vi "NumIntegrate_Rk4_K_Dbl.vi"(11 "input matrix":T1) -> (3 "output matrix":T1)   [LabVIEW 2019]
doc: "NOT DONE"
uses:
  <vilib>/Analysis/Matrix/Datatypes/RealMatrix.ctl
  <vilib>/Analysis/Matrix/NI_Matrix.lvlib
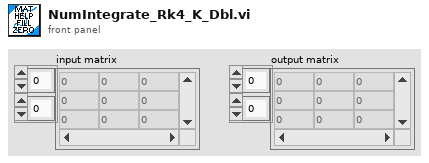
[diagram p1: front panel]
types:
  T1 = typedef "NI_Matrix.lvlib/RealMatrix.ctl" = dbl[][]
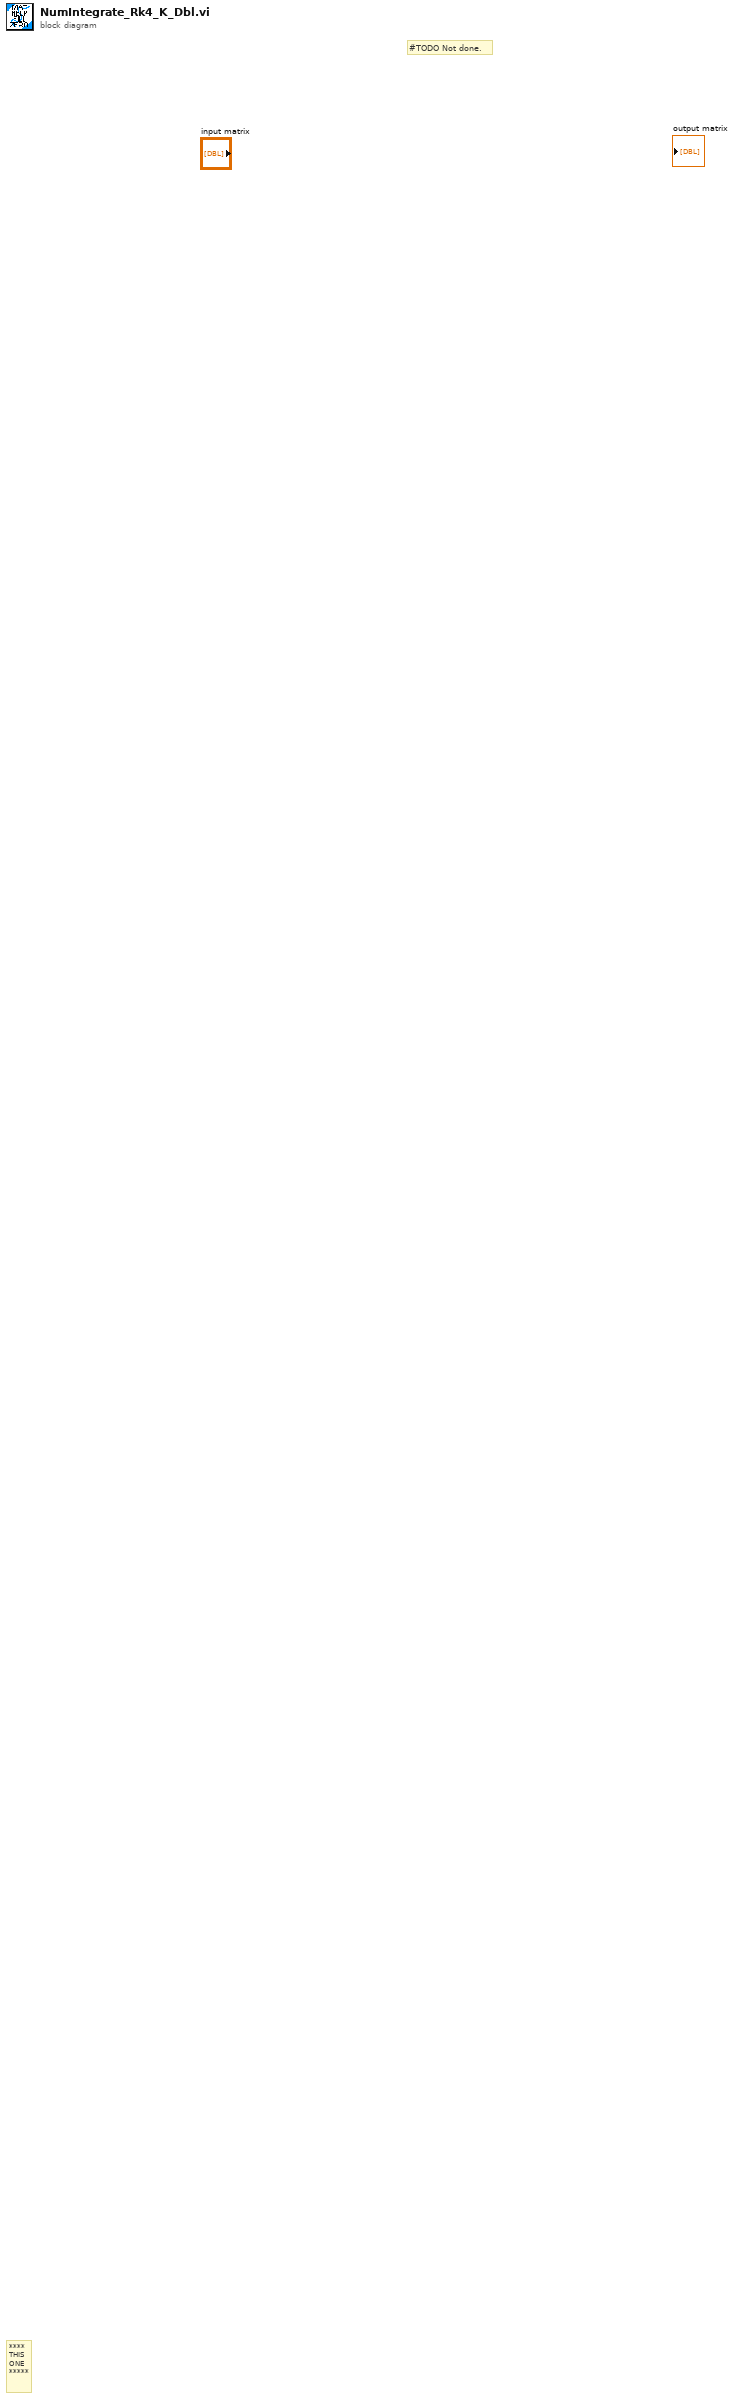
[diagram p0: block diagram]
diagram:
  # "#TODO Not done."
  # "****\nTHIS\nONE\n*****"
